vi "Ramp Time DAO.vi"(8 "error in (no error)":errorcluster, 9 "Ramp Time In":u64, 10 "Completed In":bool, 11 "Actions":T1) -> (0 "error out":errorcluster, 1 "Ramp Time Out":u64, 2 "Completed Out":bool)   [LabVIEW 2009]
uses:
  Data Access Objects/Metadata/DAO Actions.ctl
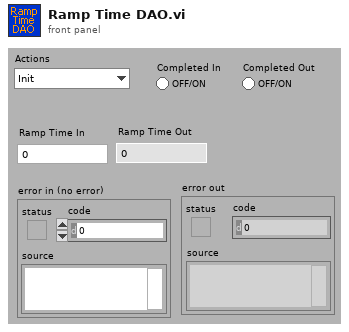
[diagram p1: front panel]
types:
  T1 = typedef "DAO Actions.ctl" = enum16{"Init", "Get", "Set"}
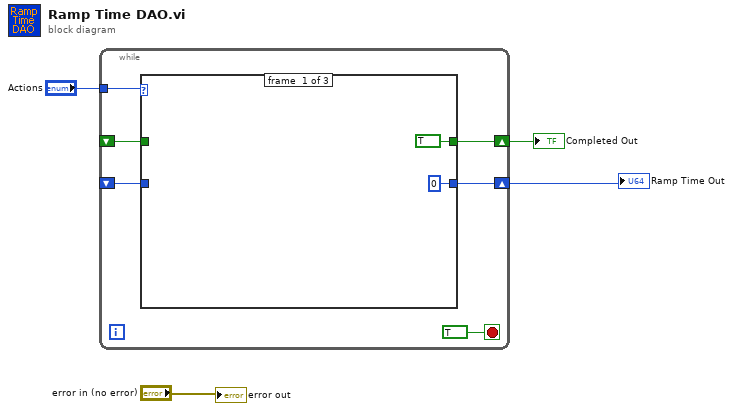
[diagram p0: block diagram]
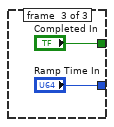
[diagram p3: hidden frame]
diagram:
  n1 = while {
    tunnel: "Actions" -> [w9]
    shift-right: [w8] -> w2
    shift-left: _ -> [w7]
    shift-right: [w6] -> w1
    shift-left: _ -> [w5]
    stop <- TRUE stop-if-true
    n2 = case shown="\"Set\"" w9 {
      tunnel: [u64 0 ("Ramp Time In") w14 "Ramp Time In"] -> w8
      tunnel: w7 -> [_ w14 _]
      tunnel: [TRUE ("Completed In") w13 "Completed In"] -> w6
      tunnel: w5 -> [_ w13 _]
      frame #0 {
      }
      frame #1 {
      }
      frame #2 {
      }
    }
  }
  "Ramp Time Out" <- w2
  "Completed Out" <- w1
  "error out" <- "error in (no error)"
